vi "Init.vi"(8 "Error In":errorcluster, 11 "reference in":refnum<class "Camera.lvclass">) -> (0 "Error Out":errorcluster, 3 "reference out":refnum<class "Camera.lvclass">)   [LabVIEW 2025, in "Camera.lvclass"]
uses:
  Camera.lvclass
  Interfaces/IConfigure/IConfigure.lvclass
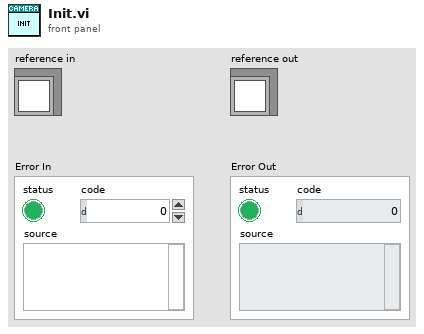
[diagram p1: front panel]
types:
  T1 = typedef "Camera.lvclass/ObjectAttributes.ctl" = cluster{"IConfigure":refnum<class "IConfigure.lvclass">, "Worker Enqueuer":refnum<class "Message Enqueuer.lvclass">, "Start Counter":i32, "Initialized":bool}
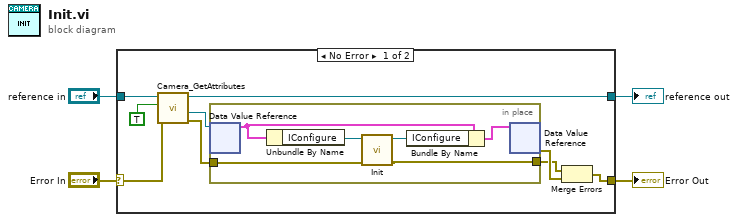
[diagram p0: block diagram]
diagram:
  n1 = case shown="No Error" "Error In" {
    selector: "Error In" -> [w13 w21]
    tunnel: [w6 w21] -> w3
    tunnel: [w11 w20] -> w1
    tunnel: "reference in" -> [w12 w20]
    frame No Error {
      n2 = call "Camera_GetAttributes.vi"("Error In"=w13, "OnlyGetDvrReference(False)"=TRUE, "reference in"=w12) -> ("Error Out"=w9:errorcluster, "DataRef"=w10:refnum<data-value>, "reference out"=w11:refnum<class "Camera.lvclass">)  [unwired: 5 in, 1 out]
      n3 = in-place {
        in-place-border: w9 -> [w15]
        in-place-border: [w14] -> w7
        n4 = in-place-dvr #1(w10) -> (w18:T1)  [unwired: 1 out]
        n5 = Unbundle By Name(w18) -> ("IConfigure"=w19:refnum<class "IConfigure.lvclass">)
        n6 = call-dynamic "Init.vi"("error in"=w15, "IInitialize in"=w19) -> ("error out"=w14:errorcluster, "IInitialize out"=w17:refnum<class "IConfigure.lvclass">)  [unwired: 8 in]
        n7 = Bundle By Name(cluster=w18, "IConfigure"=w17) -> (w16:T1)
        n8 = in-place-dvr #1(w16) -> (w8:errorcluster)  [unwired: 1 out]
      }
      n9 = Merge Errors(w7, w8) -> (w6:errorcluster)
    }
    frame Error {
    }
  }
  "Error Out" <- w3
  "reference out" <- w1
